vi "multi_final.vi"() -> ()   [LabVIEW 2023]
panel:
  out "Linear Position(mm)":dbl[](array[numeric])
  out "Motor 2 Max":dbl
  out "Motor 1 Max":dbl
  out "Force(N)":dbl[](array[numeric])
  out "Iterations":i32
  in  "Torque(Nm)":dbl[](array[numeric])
  in  "Max Torque":dbl[](array[numeric])
  in  "Velocity":dbl[](array[numeric])
  in  "Mode":T1(array[ring])
  out "Torque(Nm)":dbl[](array[numeric])
  out "Position":dbl[](array[numeric])
  out "Start Error":errorcluster
  out "Main Error":errorcluster
  in  "?":bool
  in  "Position Input":dbl[](array[slide]) min=1.5e-05 max=0.190598 step=0.1 scale=0.0..0.5
  in  "Number of Motors":i64
  # "Multi Motor Move"
  # "Telemetry"
  # "Controls"
  # "Move"
  # "Velocity Max Torque"
  # "Torque"
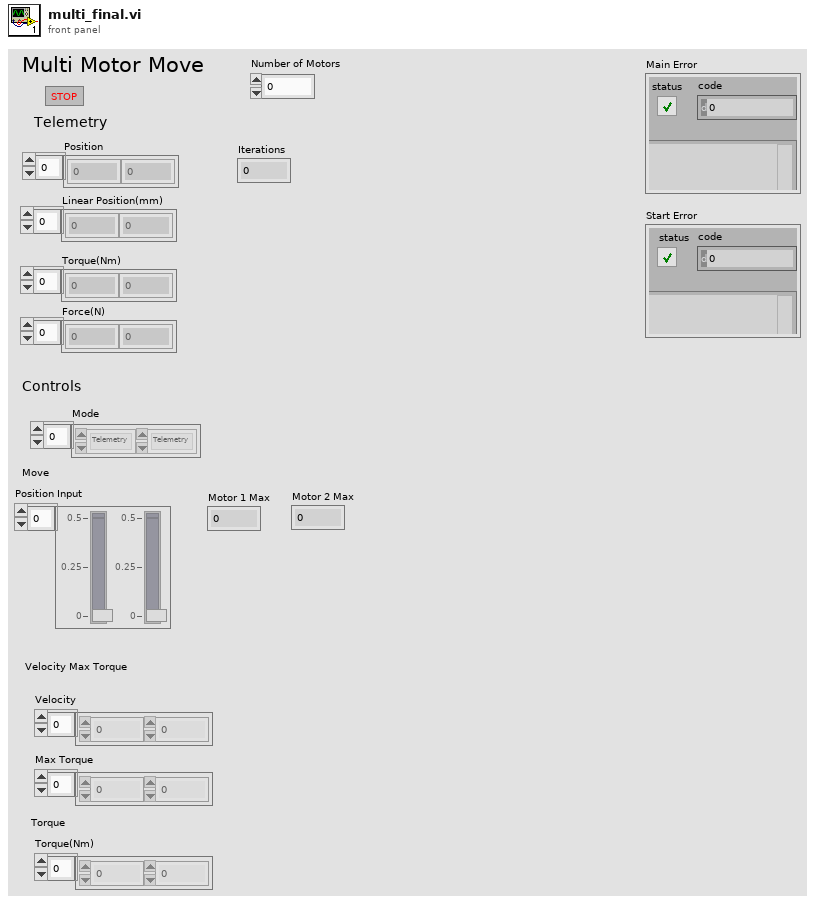
[diagram p1: front panel]
types:
  T1 = enum16{"Telemetry", "Move", "Velocity - Max Torque", "Torque"}[]
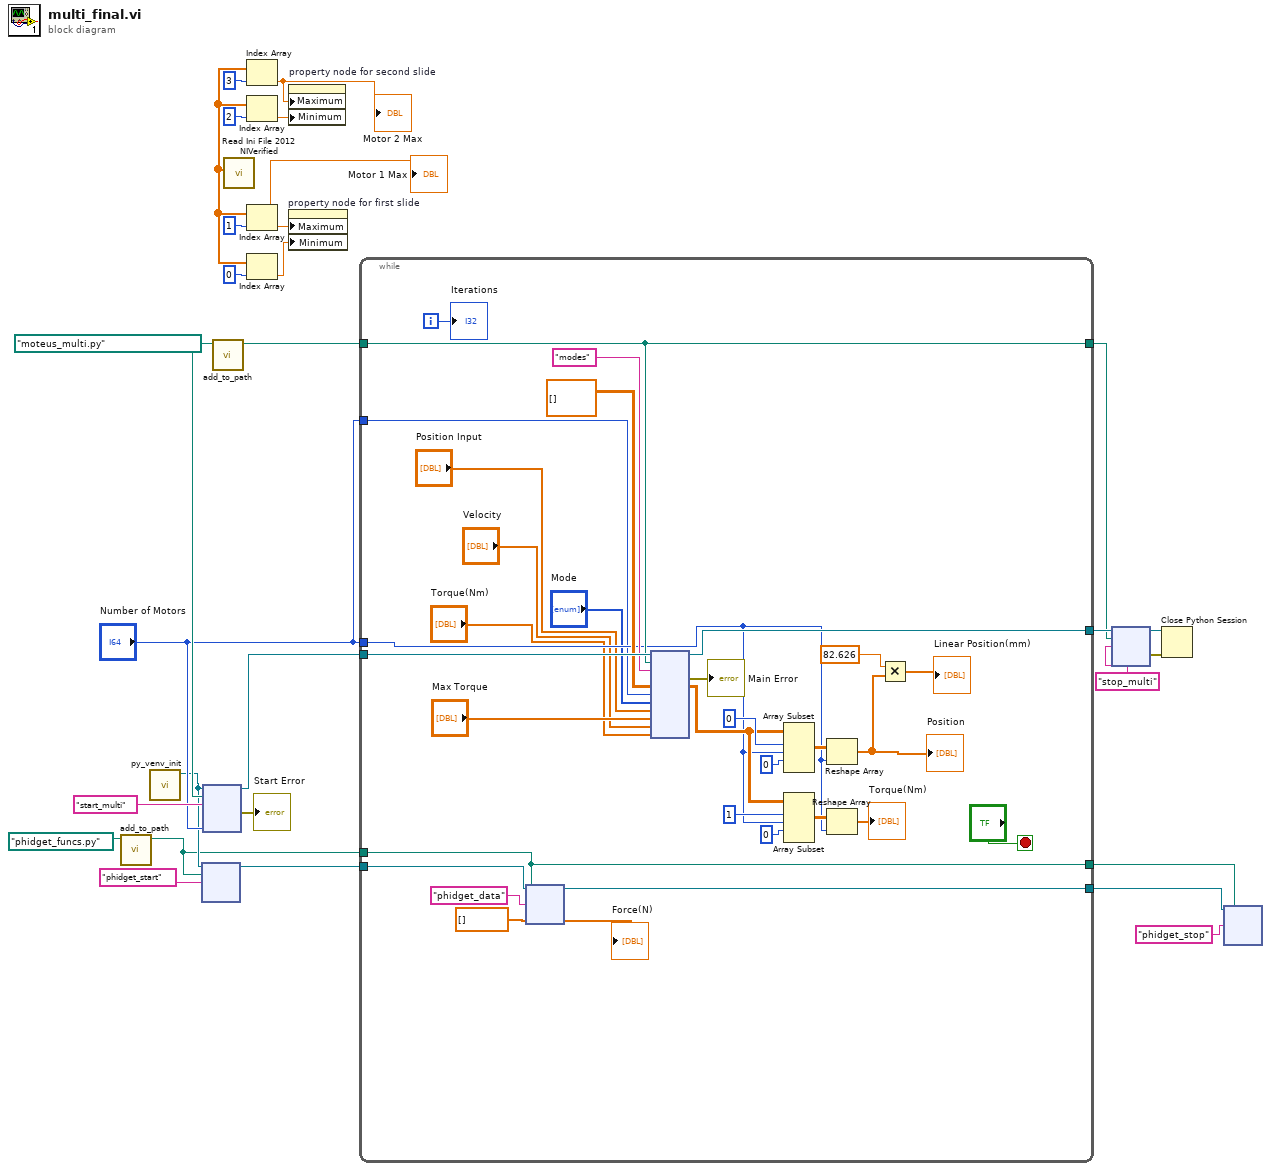
[diagram p0: block diagram]
diagram:
  n1 = call "add_to_path.vi"("Path"=path "phidget_funcs.py") -> ("appended path"=w6:path)  [unwired: 10 in]
  n2 = call "py_venv_init.vi"() -> ("Refnum out"=w8:refnum<k35>)  [unwired: 11 in]
  n3 = node(w8, w6, "phidget_start" ("function name")) -> (w7:refnum<k35>)  [unwired: 3 in, 3 out]
  n4 = call "add_to_path.vi"("Path"=path "moteus_multi.py") -> ("appended path"=w25:path)  [unwired: 10 in]
  n5 = node(w8, w25, "start_multi", "Number of Motors") -> (w26:refnum<k35>, →"Start Error":errorcluster)  [unwired: 4 in, 2 out]
  n6 = call "Read Ini File 2012 NIVerified.vi"() -> ("Array"=w12:dbl[])  [unwired: 7 in]
  n7 = Index Array(array=w12, index=3) -> (element=w1:dbl)
  "Motor 2 Max" <- w1
  n8 = Index Array(array=w12, index=2) -> (element=w14:dbl)
  n9 = Index Array(array=w12, index=1) -> (element=w2:dbl)
  "Motor 1 Max" <- w2
  n10 = Index Array(array=w12, index=0) -> (element=w16:dbl)
  n11 = property on="property node for second slide" class="Slide (strict)"("Maximum"=w1, "Minimum"=w14) -> ()  [unwired: 2 in, 2 out]
  n12 = property on="property node for first slide" class="Slide (strict)"("Maximum"=w2, "Minimum"=w16) -> ()  [unwired: 2 in, 2 out]
  n13 = while {
    tunnel: w26 -> [w60]
    tunnel: w25 -> [w55]
    tunnel: [w56] -> w24
    tunnel: [w55] -> w23
    tunnel: "Number of Motors" -> [w45]
    tunnel: "Number of Motors" -> [w44]
    tunnel: w7 -> [w35]
    tunnel: w6 -> [w33]
    tunnel: [w34] -> w4
    tunnel: [w33] -> w3
    i -> [w38]
    stop <- "?" stop-if-true
    n14 = node(w35, w33, "phidget_data" ("function name"), dbl[] []) -> (w34:refnum<k35>, →"Force(N)":dbl[])  [unwired: 1 in, 3 out]
    n15 = node(w60, w55, "modes", dbl[][] [], w44, "Mode", "Position Input", "Max Torque", "Velocity", "Torque(Nm)") -> (w56:refnum<k35>, →"Main Error":errorcluster, w51:dbl[][])  [unwired: 7 in, 2 out]
    n16 = Array Subset(array=w51, index (row)=0, length (row)=w45, index (col)=0) -> (w48:dbl[][])  [unwired: 1 in]
    n17 = Array Subset(array=w51, index (row)=1, length (row)=w45, index (col)=0) -> (w46:dbl[][])  [unwired: 1 in]
    n18 = Reshape Array(w48, w45) -> (w31:dbl[])
    "Position" <- w31
    n19 = Reshape Array(w46, w45) -> (→"Torque(Nm)":dbl[])
    n20 = Multiply(x=82.626, y=w31) -> (x*y=→"Linear Position(mm)":dbl[])
    "Iterations" <- w38
  }
  n21 = node(w24, w23, "stop_multi") -> (w20:refnum<k35>, w19:errorcluster)  [unwired: 3 in, 2 out]
  n22 = Close Python Session(session in=w20, error in=w19) -> ()  [unwired: 1 out]
  n23 = node(w4, w3, "phidget_stop" ("function name")) -> ()  [unwired: 3 in, 4 out]
